vi "keithley-2450_j-t_list.vi"(0 "VISA resource name in":refnum<visa-resource-name>, 1 "Shutter open?":bool, 11 "error in (no error)":errorcluster, 12 "Voltage List":dbl[](array[numeric])) -> (4 "VISA resource name out":refnum<visa-resource-name>, 6 "Data Array":dbl[][](array[numeric]), 15 "Measurement Complete":bool)   [LabVIEW 2016]
doc: "Configures a sweep and takes voltage and current readings at each point."
uses:
  <instrlib>/Keithley 2450/Keithley 2450.lvlib
panel:
  in  "Source Mode  (0: Voltage)":u16(ring) items=["Voltage", "Current"]
  # "(c) 2006 National Instruments.  ALL RIGHTS RESERVED."
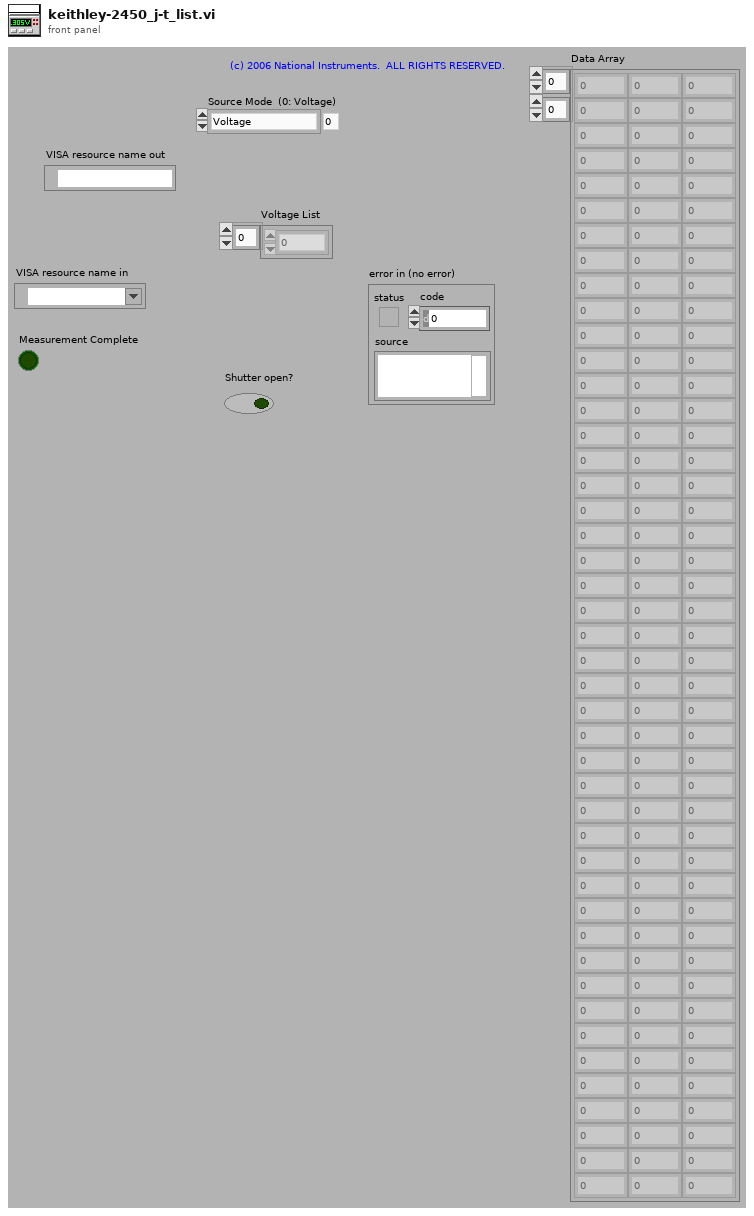
[diagram p1: front panel]
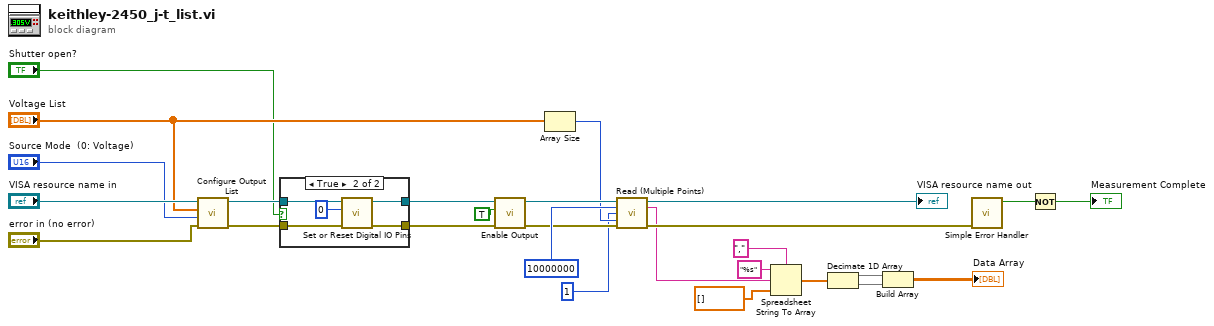
[diagram p0: block diagram]
diagram:
  n1 = call <instrlib>:"Configure Output List.vi"("error in (no error)"="error in (no error)", "Source Mode  (0: Voltage)"="Source Mode  (0: Voltage)", "Output List"="Voltage List", "VISA resource name"="VISA resource name in") -> ("error out"=w17:errorcluster, "VISA resource name out"=w18:refnum<visa-resource-name>)  [unwired: 6 in]
  n2 = case shown="True" "Shutter open?" {
    tunnel: w18 -> [w29 w33]
    tunnel: w17 -> [w28 w32]
    tunnel: [w29 w31] -> w16
    tunnel: [w28 w30] -> w15
    frame False {
    }
    frame True {
      n3 = call <instrlib>:"Set or Reset Digital IO Pins.vi"("error in (no error)"=w32, "Digital IO Line (1)"=0, "VISA resource name"=w33) -> ("error out"=w30:errorcluster, "VISA resource name out"=w31:refnum<visa-resource-name>)  [unwired: 7 in]
    }
  }
  n4 = call <instrlib>:"Enable Output.vi"("error in (no error)"=w15, "Enable Output (T: Enable)"=TRUE ("Output (Off)"), "VISA resource name"=w16) -> ("error out"=w13:errorcluster, "VISA resource name out"=w14:refnum<visa-resource-name>)  [unwired: 7 in]
  n5 = Array Size(array="Voltage List") -> (size(s)=w10:i32)
  n6 = call <instrlib>:"Read (Multiple Points).vi"("VISA resource name"=w14, "Timeout (10000 ms)"=10000000, "Start Index (1)"=1, "End Index (1)"=w10, "error in (no error)"=w13) -> ("VISA resource name out"=→"VISA resource name out":refnum<visa-resource-name>, "Data out"=w2:string, "error out"=w27:errorcluster)  [unwired: 8 in]
  n7 = Spreadsheet String To Array(delimiter (Tab)=",", format string="%s", spreadsheet string=w2, array type (2D Dbl)=dbl[] []) -> (array=w5:dbl[])
  n8 = Decimate 1D Array(w5) -> (w4:dbl[], w3:dbl[])
  n9 = Build Array(w4, w3) -> (→"Data Array":dbl[][])
  n10 = call <vilib>:"Simple Error Handler.vi"("error in (no error)"=w27) -> ("error?"=w25:bool)  [unwired: 4 in, 4 out]
  n11 = Not(x=w25) -> (.not. x?=→"Measurement Complete":bool)
